vi "Delete Element.vi"(8 "error in (no error)":errorcluster, 9 "Variant":variant, 10 "Key":string, 11 "SMO.Dictionary.Variant in":refnum<class "SMO.Dictionary.Variant.lvclass">) -> (0 "error out":errorcluster, 1 "Deleted Element":T1, 3 "SMO.Dictionary.Variant out":refnum<class "SMO.Dictionary.Variant.lvclass">)   [LabVIEW 2013, in "SMO.Dictionary.lvlib" / "SMO.Dictionary.Variant.lvclass"]
uses:
  SMO.Dictionary.Variant.lvclass
  SMO.Dictionary/Typedefs/PrivateEvents--SMO.Dictionary.KeyValue-Pair.ctl
  SMO.Dictionary.Variant.lvclass/SMO.Dictionary.Variant.ctl
  SMO.Dictionary/SMO.Dictionary.lvclass
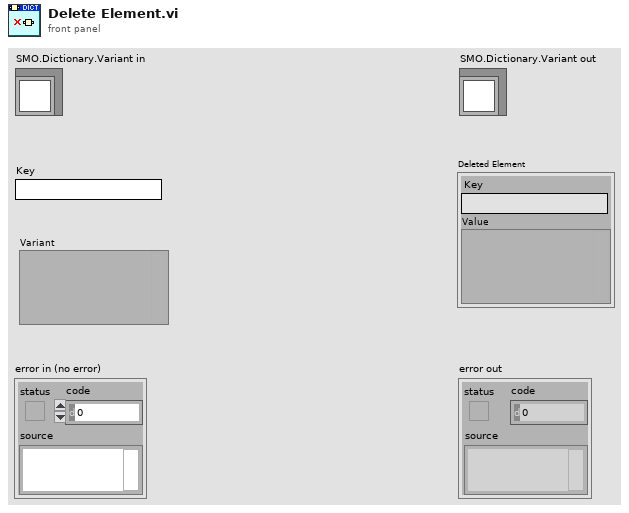
[diagram p1: front panel]
types:
  T1 = typedef "SMO.Dictionary.lvlib/SMO.Dictionary.lvclass/PrivateEvents--SMO.Dictionary.KeyValue-Pair.ctl" = cluster{"Key":string, "Value":variant}
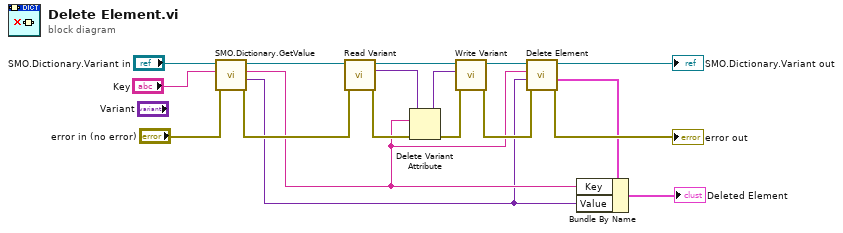
[diagram p0: block diagram]
diagram:
  n1 = call "SMO.Dictionary.GetValue.vi"("error in (no error)"="error in (no error)", "Key"="Key", "SMO.Dictionary"="SMO.Dictionary.Variant in") -> ("error out"=w10:errorcluster, "Value"=w1:variant, "Key"=w3:string, "SMO.Dictionary out"=w13:refnum<class "SMO.Dictionary.Variant.lvclass">)  [unwired: 4 in, 1 out]
  n2 = call "Read Variant.vi"("error in (no error)"=w10, "SMO.Dictionary.Variant in"=w13) -> ("error out"=w9:errorcluster, "Variant"=w12:variant, "SMO.Dictionary.Variant out"=w14:refnum<class "SMO.Dictionary.Variant.lvclass">)  [unwired: 7 in]
  n3 = Delete Variant Attribute(4:w9, 6:w3, 7:w12) -> (0:w8:errorcluster, 3:w11:variant)  [unwired: 1 out]
  n4 = call "Write Variant.vi"("error in (no error)"=w8, "Variant"=w11, "SMO.Dictionary.Variant in"=w14) -> ("error out"=w5:errorcluster, "SMO.Dictionary.Variant out"=w7:refnum<class "SMO.Dictionary.Variant.lvclass">)  [unwired: 7 in]
  n5 = call-parent "Delete Element.vi"("error in (no error)"=w5, "Variant"=w1, "Key"=w3, "SMO.Dictionary in"=w7) -> ("error out"=→"error out":errorcluster, "Deleted Element"=w2:T1, "SMO.Dictionary out"=→"SMO.Dictionary.Variant out":refnum<class "SMO.Dictionary.Variant.lvclass">)  [unwired: 5 in]
  n6 = Bundle By Name(cluster=w2, "Key"=w3, "Value"=w1) -> (→"Deleted Element":T1)
